vi "fpga_LP2 Process.vi"(0 "re":fxp<+/-,32,5> format="%.29g", 1 "reset":bool, 5 "im":fxp<+/-,32,5> format="%.29g", 7 "#Ch":fxp<+,5,5>=16.0, 9 "input valid":bool, 12 "ready for output":bool) -> (4 "re filtered":fxp<+/-,32,6> format="%.28g", 6 "im filtered":fxp<+/-,32,6> format="%.28g", 10 "output valid":bool, 14 "ready for input":bool)   [LabVIEW 2011, in "NI_EP_PMU_FPGA.lvlib"]
uses:
  <vilib>/addons/Electrical Power/PMU/NI_EP_PMU_FPGA.lvlib
  <vilib>/rvi/FXPMathLib/basic elements/FxpDiscreteDelay/XNode/nifxpmath_DiscreteDelay.xnode
  <vilib>/addons/Electrical Power/PQ/Resampling/NI_EP_Resample_FPGA.lvlib
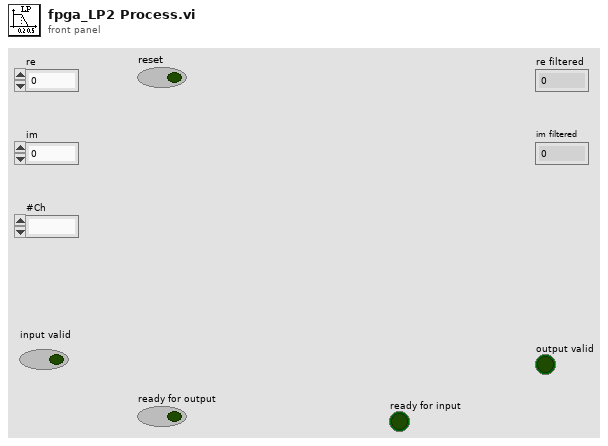
[diagram p1: front panel]
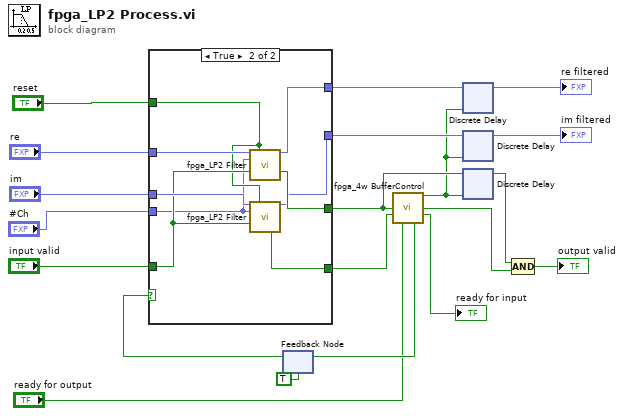
[diagram p0: block diagram]
diagram:
  n1 = feedback #1(TRUE ("logic enable")) -> (w15:bool)
  n2 = case shown="True" w15 {
    tunnel: "input valid" -> [_ w27]
    tunnel: "reset" -> [_ w22]
    tunnel: [_ w26] -> w7
    tunnel: [_ w23] -> w18
    tunnel: [_ w25] -> w3
    tunnel: [_ w24] -> w5
    tunnel: "re" -> [_ w29]
    tunnel: "im" -> [_ w28]
    tunnel: "#Ch" -> [_ w21]
    frame False {
    }
    frame True {
      n3 = call <vilib>:"fpga_LP2 Filter.vi"("input data"=w29, "reset"=w22, "#Ch"=w21, "input valid"=w27) -> ("output data"=w25:fxp<+/-,32,6>, "output valid"=w26:bool)  [unwired: 9 in, 1 out]
      n4 = call <vilib>:"fpga_LP2 Filter.vi"("input data"=w28, "reset"=w22, "#Ch"=w21, "input valid"=w27) -> ("output data"=w24:fxp<+/-,32,6>, "ready for input"=w23:bool)  [unwired: 9 in, 1 out]
    }
  }
  n5 = call <vilib>:"fpga_4w BufferControl.vi"("DR"=w7, "RFI"=w18, "RFO"="ready for output") -> ("buff enable"=w2:bool, "output valid"=w17:bool, "ready for input"=→"ready for input":bool, "logic enable"=w16:bool)  [unwired: 9 in]
  n6 = feedback-in #1(w16) -> ()
  n7 = xnode "Discrete Delay"("D"=w3, "enable"=w2) -> ("Q"=→"re filtered":fxp<+/-,32,6>)
  n8 = xnode "Discrete Delay"("D"=w5, "enable"=w2) -> ("Q"=→"im filtered":fxp<+/-,32,6>)
  n9 = xnode "Discrete Delay"("D"=w7, "enable"=w2) -> ("Q"=w6:bool)
  n10 = Compound Arithmetic op=AND(w6, w17) -> (→"output valid":bool)
